vi "Save Error Message.vi"(8 "error in (no error)":errorcluster, 10 "String":string, 11 "Path":path) -> (0 "error out":errorcluster)   [LabVIEW 2020, in "Error Handler.lvlib"]
uses:
  Error Handler.lvlib
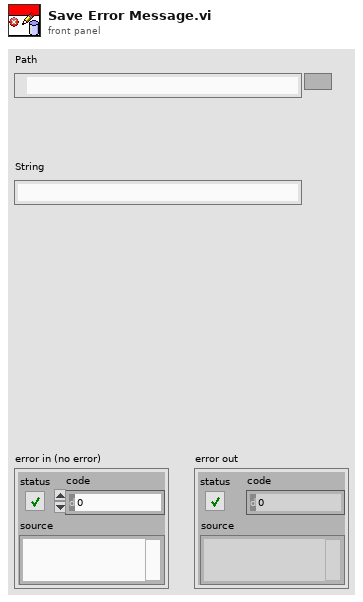
[diagram p1: front panel]
types:
  T1 = enum16{"open", "replace", "create", "open or create", "replace or create", "replace or create with confirmation"}
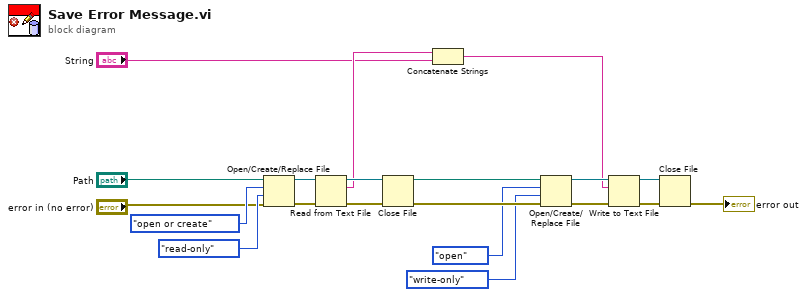
[diagram p0: block diagram]
diagram:
  n1 = Open/Create/Replace File(file path (use dialog)="Path", error in="error in (no error)", operation (0:open)=T1."open or create", access (0:read/write)=enum16{"read/write", "read-only", "write-only"}."read-only") -> (refnum out=w20:refnum<file>, error out=w19:errorcluster)  [unwired: 2 in, 1 out]
  n2 = Read from Text File(file (use dialog)=w20, error in=w19) -> (refnum out=w18:refnum<file>, text=w6:string, error out=w17:errorcluster)  [unwired: 2 in, 1 out]
  n3 = Close File(refnum=w18, error in=w17) -> (path=w14:path, error out=w13:errorcluster)
  n4 = Concatenate Strings(w6, "String") -> (w2:string)
  n5 = Open/Create/Replace File(file path (use dialog)=w14, error in=w13, operation (0:open)=T1."open", access (0:read/write)=enum16{"read/write", "read-only", "write-only"}."write-only") -> (refnum out=w12:refnum<file>, error out=w15:errorcluster)  [unwired: 2 in, 1 out]
  n6 = Write to Text File(file (use dialog)=w12, text=w2, error in=w15) -> (refnum out=w11:refnum<file>, error out=w16:errorcluster)  [unwired: 1 in, 1 out]
  n7 = Close File(refnum=w11, error in=w16) -> (error out=→"error out":errorcluster)  [unwired: 1 out]
